vi "UDP模拟量发送数据位置.vi"(1 "数据区字长":u16, 2 "报文类型":u16, 3 "发送方标识":u16) -> ()   [LabVIEW 2010]
uses:
  全局量/全局_配置.vi
panel:
  in  "第几个":u16
  in  "第几组":u16
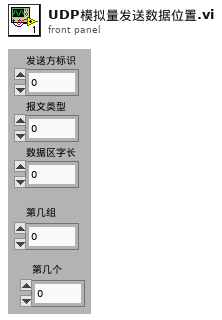
[diagram p1: front panel]
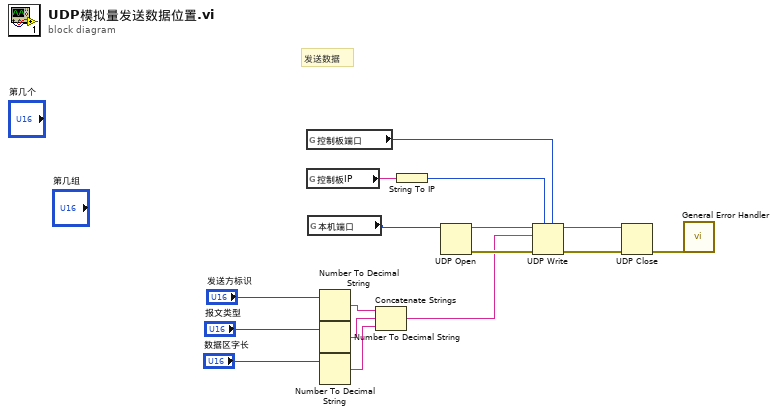
[diagram p0: block diagram]
diagram:
  # "发送数据"
  n1 = global read "全局_配置.vi" "控制板端口"() -> (w10:u16)
  n2 = global read "全局_配置.vi" "控制板IP"() -> (w9:string)
  n3 = global read "全局_配置.vi" "本机端口"() -> (w8:u16)
  n4 = Number To Decimal String(number="发送方标识") -> (decimal integer string=w4:string)  [unwired: 1 in]
  n5 = Number To Decimal String(number="报文类型") -> (decimal integer string=w3:string)  [unwired: 1 in]
  n6 = Number To Decimal String(number="数据区字长") -> (decimal integer string=w2:string)  [unwired: 1 in]
  n7 = Concatenate Strings(w4, w3, w2) -> (w1:string)
  n8 = String To IP(1:w9) -> (0:w11:u32)
  n9 = UDP Open(11:w8) -> (port=w16:refnum<k16>, 0:w15:errorcluster)  [unwired: 4 in, 1 out]
  n10 = UDP Write(address=w11, port or service name=w10, connection ID=w16, data in=w1, 8:w15) -> (error out=w12:errorcluster, 3:w13:refnum<k16>)  [unwired: 1 in]
  n11 = UDP Close(connection ID=w13, 8:w12) -> (error out=w14:errorcluster)  [unwired: 1 out]
  n12 = call <vilib>:"General Error Handler.vi"("error in (no error)"=w14) -> ()  [unwired: 10 in, 5 out]
